vi "Example XYGraph Peaks&Valleys.vi"() -> ()   [LabVIEW 2015]
uses:
  controls/PeaksValleyOptions.ctl
  <vilib>/ptbypt/NI_PtbyPt.lvlib
panel:
  in  "Peaks and Valleys":T1={"Peaks"={"#"=50, "size"=7, "WidthThreshold"=3, "AmplitudeThreshold"=0.0, "Fill"=TRUE, "PlotIndexes (All)"=[]}, "Valleys"={"#"=50, "size"=7, "WidthThreshold"=3, "AmplitudeThreshold"=0.0, "Fill"=TRUE, "PlotIndexes (All)"=[]}} {"Valleys"."AmplitudeThreshold" min=0.0 format="%.3f"; "Valleys"."WidthThreshold" min=3; "Valleys"."size" min=1 max=50; "Peaks"."AmplitudeThreshold" min=0.0 format="%.3f"; "Peaks"."WidthThreshold" min=3; "Peaks"."size" min=1 max=50}
  out "XY Graph":cluster{dbl[], dbl[]}[](graph)
  # "Instructions: Move the mouse over the graphs, and adjust any of the options at the right. to see the effect."
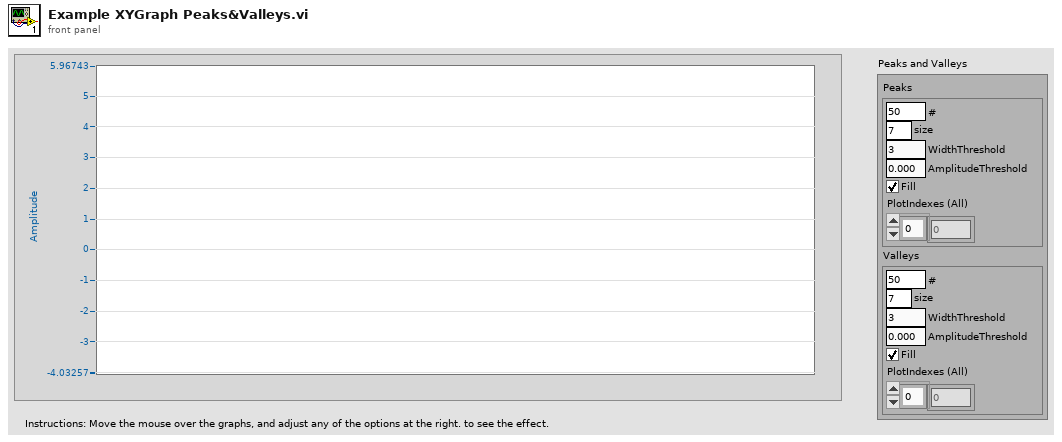
[diagram p1: front panel]
types:
  T1 = typedef "PeaksValleyOptions.ctl" = cluster{"Peaks":cluster{"#":i32, "size":i16, "WidthThreshold":i32, "AmplitudeThreshold":dbl, "Fill":bool, "PlotIndexes (All)":u16[]}, "Valleys":cluster{"#":i32, "size":i16, "WidthThreshold":i32, "AmplitudeThreshold":dbl, "Fill":bool, "PlotIndexes (All)":u16[]}}
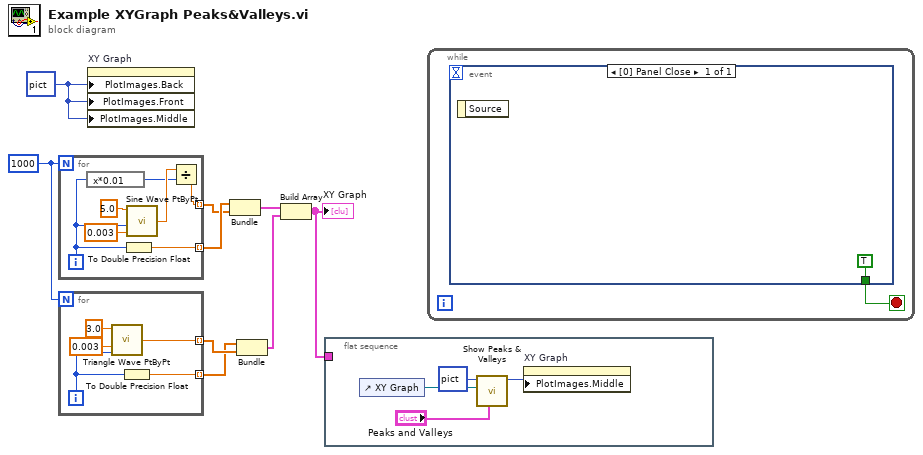
[diagram p0: block diagram]
diagram:
  w2 = picture data[5B] ("Plot Images:Back")
  w3 = 1000
  n1 = for {
    N: w3 -> [_]
    tunnel: [w11] -> w8 mode=indexing
    tunnel: [w16] -> w9 mode=indexing
    i -> [w13]
    w14 = 0.003 ("frequency")
    n2 = expression code="x*0.01"(w13) -> (w10:i32)
    n3 = To Double Precision Float(number=w13) -> (double precision float=w16:dbl)
    n4 = call <vilib>:"Sine Wave PtByPt.vi"("time"=w14, "phase"=w13, "frequency"=w14, "amplitude"=5.0) -> ("sine wave"=w12:dbl)
    n5 = Divide(x=w12, y=w10) -> (x/y=w11:dbl)
  }
  n6 = for {
    N: w3 -> [_]
    tunnel: [w21] -> w6 mode=indexing
    tunnel: [w17] -> w5 mode=indexing
    i -> [w20]
    n7 = call <vilib>:"Triangle Wave PtByPt.vi"("time"=w20, "frequency"=0.003, "amplitude"=3.0) -> ("triangle wave"=w21:dbl)  [unwired: 1 in]
    n8 = To Double Precision Float(number=w20) -> (double precision float=w17:dbl)
  }
  n9 = property on="XY Graph" class="XYGraph (strict)"("PlotImages.Back"=w2, "PlotImages.Front"=w2, "PlotImages.Middle"=w2) -> ()  [unwired: 2 in, 2 out]
  n10 = Bundle(w9, w8) -> (w7:cluster{dbl[], dbl[]})  [unwired: 1 in]
  n11 = Bundle(w5, w6) -> (w4:cluster{dbl[], dbl[]})  [unwired: 1 in]
  n12 = Build Array(w7, w4) -> (w1:cluster{dbl[], dbl[]}[])
  "XY Graph" <- w1
  n13 = flat-sequence {
    tunnel: w1 -> [_]
    frame #0 {
      n14 = control-ref of="XY Graph"() -> (w25:refnum<vi>)
      n15 = call "Show Peaks & Valleys.vi"("peaksValleysOptions"="Peaks and Valleys", "XY Graph"=w25, "input picture"=picture data[5B]) -> ("output picture"=w24:picture)  [unwired: 7 in, 1 out]
      n16 = property on="XY Graph" class="XYGraph (strict)"("PlotImages.Middle"=w24) -> ()  [unwired: 2 in, 2 out]
    }
  }
  n17 = while {
    stop <- w26 stop-if-true
    n18 = event shown="[0] Panel Close" {
      selector: _ -> [_]
      dyn-events: _ -> [_]
      timeout: _ -> [_]
      tunnel: [TRUE] -> w26
      event Panel Close {
        n19 = event-data() -> ()  [unwired: 1 in, 1 out]
      }
    }
  }
